vi "LabVIEW HOGv2.0.vi"() -> ()   [LabVIEW 2014]
uses:
  <vilib>/Instr/_visa.llb/VISA Configure Serial Port (Instr).vi
panel:
  in  "stop":bool
  in  "Motor control":bool
  in  "Servo2":dbl(slide) scale=0.0..10.0
  in  "Servo1":dbl(slide) scale=0.0..10.0
  in  "baud rate":u32=9600
  in  "Select COM port":refnum<visa-resource-name>
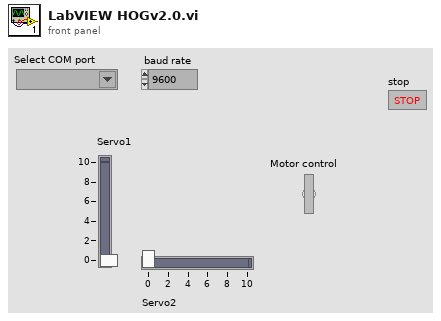
[diagram p1: front panel]
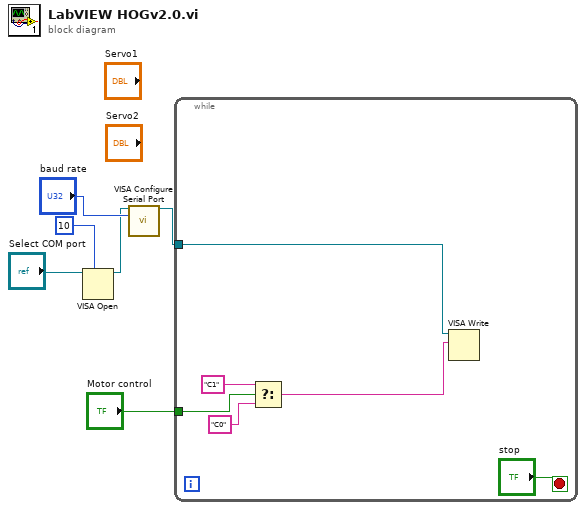
[diagram p0: block diagram]
diagram:
  n1 = VISA Open(timeout (0)=u32 10 ("VISA Open timeout (0)"), VISA resource name="Select COM port") -> (VISA resource name=w2:refnum<visa-resource-name>)  [unwired: 3 in, 1 out]
  n2 = call-poly "VISA Configure Serial Port"("VISA resource name"=w2, "baud rate (9600)"="baud rate") -> ("VISA resource name out"=w5:refnum<visa-resource-name>)  [unwired: 12 in, 1 out]
  n3 = while {
    tunnel: "Motor control" -> [w10]
    tunnel: w5 -> [w9]
    stop <- "stop" stop-if-true
    n4 = Select(t="C1", s=w10, f="C0") -> (s? t:f=w7:string)
    n5 = VISA Write(VISA resource name=w9, write buffer=w7) -> ()  [unwired: 1 in, 3 out]
  }
